vi "sv_Resample Filter Prototype Design.vi"(10 "rolloff":dbl) -> (3 "filter prototype out":T1={"left wing"=[], "increment"=[], "max dec"=128, "timing jitter"=enum."Interpolation", "band limiting?"=TRUE} {"increment" format="%.2f"; "left wing" format="%.2f"})   [LabVIEW 2017, in "SoundVib_Resampling.lvlib"]
doc: "Design a filter prototype for arbitrary resampling."
uses:
  <vilib>/addons/Sound and Vibration/Order Analysis/Resample Order Tracking/SoundVib_Resampling.lvlib
  <vilib>/addons/_NISVFA/_Shared subVIs/Controls/OAT Resample Filter Prototype.ctl
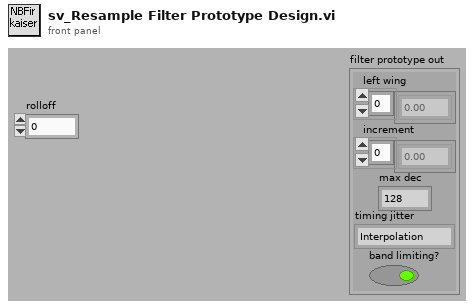
[diagram p1: front panel]
types:
  T1 = typedef "OAT Resample Filter Prototype.ctl" = cluster{"left wing":dbl[], "increment":dbl[], "max dec":i32, "timing jitter":enum32{"Interpolation", "Rounding"}, "band limiting?":bool}
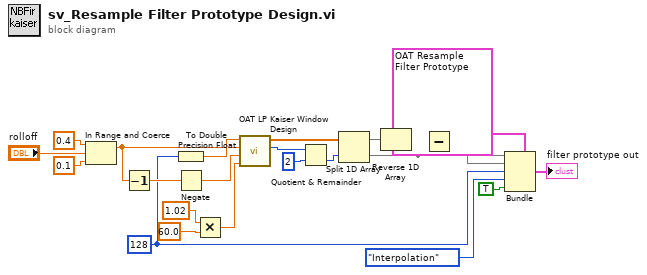
[diagram p0: block diagram]
diagram:
  w5 = 128 ("maximum decimation\nfactor (auto)")
  n1 = In Range and Coerce(upper limit=0.4, x="rolloff", lower limit=0.1 ("y")) -> (coerced(x)=w1:dbl)  [unwired: 1 out]
  n2 = Decrement(x=w1) -> (x-1=w12:dbl)
  n3 = To Double Precision Float(number=w5) -> (double precision float=w4:dbl)
  n4 = Negate(x=w12) -> (-x=w11:dbl)
  n5 = Multiply(x=1.02, y=60.0) -> (x*y=w8:dbl)
  n6 = call <vilib>:"OAT LP Kaiser Window Design.vi"("A stop [dB]"=w8, "stopband"=w11, "passband"=w1, "fs"=w4) -> ("taps"=w19:i32, "filter coefficients"=w21:dbl[])  [unwired: 5 in, 1 out]
  n7 = Quotient & Remainder(x=w19, y=2) -> (floor(x/y)=w20:i32)  [unwired: 1 out]
  n8 = Split 1D Array(array=w21, index=w20) -> (first subarray=w17:dbl[], second subarray=w13:dbl[])
  n9 = Reverse 1D Array(array=w17) -> (reversed array=w14:dbl[])
  n10 = Subtract(x=w14, y=w13) -> (x-y=w16:dbl[])
  n11 = Bundle(cluster=T1 {"left wing"=array[915 elements], "increment"=array[914 elements], "max dec"=128, "timing jitter"=enum."Interpolation", "band limiting?"=TRUE} ("filter prototype"), "left wing"=w13, "increment"=w16, "max dec"=w5, "timing jitter"=enum32{"Interpolation", "Rounding"}."Interpolation", "band limiting?"=TRUE) -> (→"filter prototype out":T1)
